vi "Read formatted request string.vi"(8 "error in (no error)":errorcluster, 11 "Request in":refnum<class "Request.lvclass">) -> (0 "error out":errorcluster, 2 "formatted request string":string, 3 "Request out":refnum<class "Request.lvclass">)   [LabVIEW 2016, in "Request.lvclass"]
uses:
  Request.lvclass
  C:/Users/tblair/Documents/Git Projects/JSONRPC/Source/Classes/JSONable/JSONable.lvclass
  JSONable/JSONable.lvclass
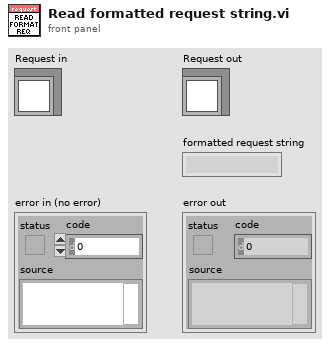
[diagram p1: front panel]
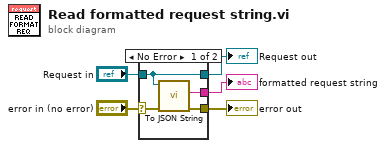
[diagram p0: block diagram]
diagram:
  n1 = case shown="No Error" "error in (no error)" {
    selector: "error in (no error)" -> [w7 w11]
    tunnel: [w6 w11] -> w4
    tunnel: [w9 w10] -> w2
    tunnel: "Request in" -> [w9 w10]
    tunnel: [w8 _] -> w1
    frame No Error {
      n2 = call "To JSON String.vi"("error in (no error)"=w7, "JSONable in"=w9) -> ("error out"=w6:errorcluster, "JSON String"=w8:string)  [unwired: 7 in, 1 out]
    }
    frame Error {
    }
  }
  "error out" <- w4
  "Request out" <- w2
  "formatted request string" <- w1
